vi "getAsDictionary.vi"(8 "error in (no error)":errorcluster, 11 "IStruct in":refnum<class "IStruct.lvclass">) -> (0 "error out":errorcluster, 2 "Dict out":refnum<class "IDict.lvclass">, 3 "IStruct out":refnum<class "IStruct.lvclass">)   [LabVIEW 2022 SP3, in "openDAQ.lvlib" / "daqCoreTypes.lvlib" / "IStruct.lvclass"]
uses:
  <instrlib>/openDAQ/Public/Classes/daqCoreTypes/IStruct/IStruct.lvclass
  <instrlib>/openDAQ/Public/Classes/daqCoreTypes/IStruct/IStruct.lvclass/IStruct.ctl
  <instrlib>/openDAQ/Public/Classes/daqCoreTypes/IDict/IDict.lvclass
  <instrlib>/openDAQ/Binaries/Windows/x86/copendaq32.dll
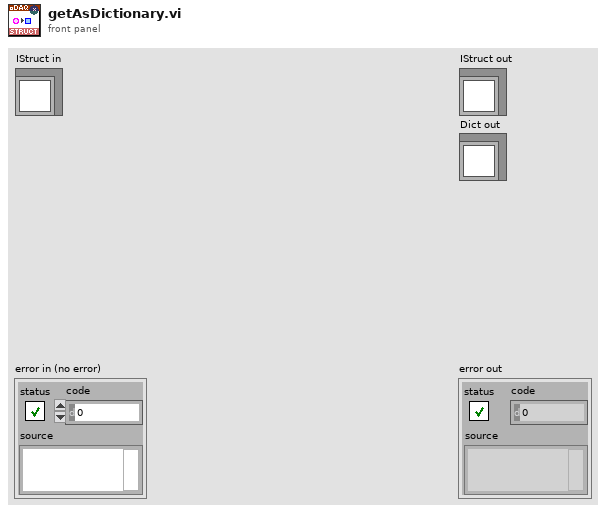
[diagram p1: front panel]
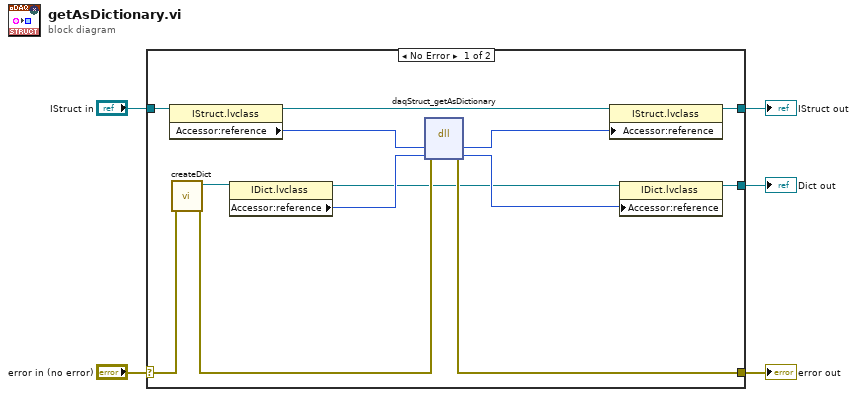
[diagram p0: block diagram]
diagram:
  n1 = case shown="No Error" "error in (no error)" {
    selector: "error in (no error)" -> [w13 w20]
    tunnel: [w9 w20] -> w4
    tunnel: [w15 w19] -> w2
    tunnel: "IStruct in" -> [w18 w19]
    tunnel: [w6 _] -> w1
    frame No Error {
      n2 = property class="IStruct.lvclass"(reference=w18) -> (reference out=w16:refnum<class "IStruct.lvclass">, "Accessor:reference"=w17:i64)  [unwired: 1 in, 1 out]
      n3 = call <instrlib>:"createDict.vi"("error in (no error)"=w13) -> ("error out"=w12:errorcluster, "IDict out"=w11:refnum<class "IDict.lvclass">)  [unwired: 9 in]
      n4 = property class="IDict.lvclass"(reference=w11) -> (reference out=w7:refnum<class "IDict.lvclass">, "Accessor:reference"=w10:i64)  [unwired: 1 in, 1 out]
      n5 = dll-call lib="C:/Program Files (x86)/National Instruments/LabVIEW 2022/instr.lib/openDAQ/Binaries/Windows/x86/copendaq*.*" fn="daqStruct_getAsDictionary"(error in=w12, "struct"=w17, "dict"=w10) -> (error out=w9:errorcluster, "struct"=w14:i64, "dict"=w8:i64)  [unwired: 3 in, 1 out]
      n6 = property class="IStruct.lvclass"(reference=w16, "Accessor:reference"=w14) -> (reference out=w15:refnum<class "IStruct.lvclass">)  [unwired: 1 in, 1 out]
      n7 = property class="IDict.lvclass"(reference=w7, "Accessor:reference"=w8) -> (reference out=w6:refnum<class "IDict.lvclass">)  [unwired: 1 in, 1 out]
    }
    frame Error {
    }
  }
  "error out" <- w4
  "IStruct out" <- w2
  "Dict out" <- w1
